vi "Init Aurora.vi"(8 "error in (no error)":errorcluster, 11 "Aurora COM Port":T1=enum."COM4") -> (0 "error out":errorcluster, 2 "Aurora Connected?":bool, 3 "Frame Grabber Data":T2)   [LabVIEW 2017]
uses:
  Controls/Tracking Data.ctl
  Controls/Packet Data.ctl
  Controls/Rigid Body Info.ctl
  Controls/Position.ctl
  Controls/Orientation.ctl
  Controls/Tracker Type.ctl
  Controls/COM Port.ctl
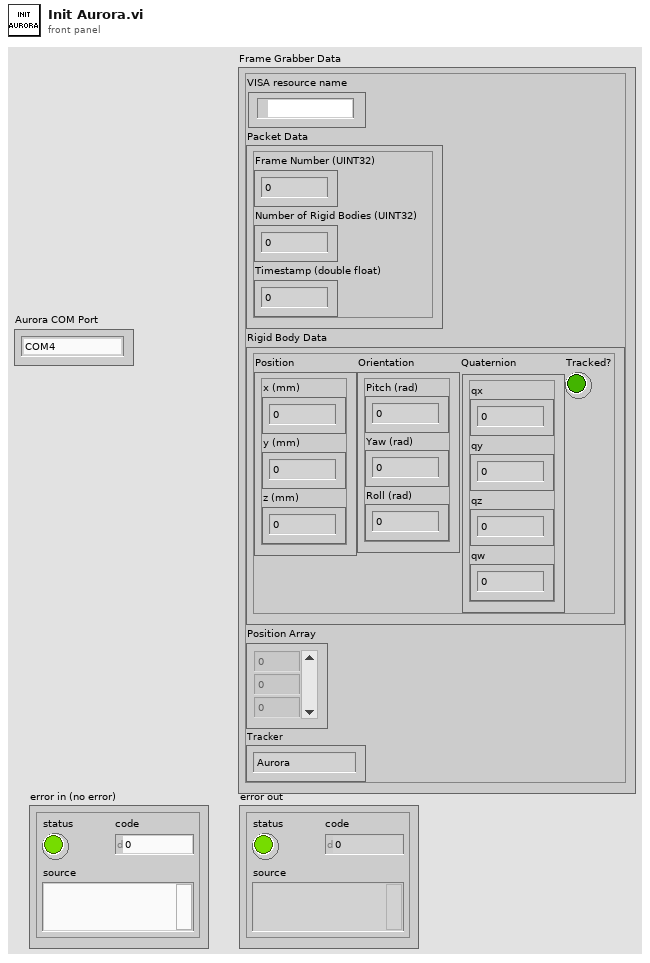
[diagram p1: front panel]
types:
  T1 = typedef "COM Port.ctl" = enum16{"COM1", "COM2", "COM3", "COM4", "COM5", "COM6", "COM7", "COM8", "COM9", "COM10", "COM11", "COM12", "COM13", "COM14", "COM15", "COM16", "COM17", "COM18", "COM19", "COM20"}
  T2 = typedef "Tracking Data.ctl" = cluster{"VISA resource name":refnum<visa-resource-name>, "Packet Data":T3, "Rigid Body Data":T4, "Position Array":dbl[][], "Tracker":T7}
  T3 = typedef "Packet Data.ctl" = cluster{"Frame Number (UINT32)":u32, "Number of Rigid Bodies (UINT32)":u32, "Timestamp (double float)":dbl}
  T4 = typedef "Rigid Body Info.ctl" = cluster{"Position":T5, "Orientation":T6, "Quaternion":cluster{"qx":sgl, "qy":sgl, "qz":sgl, "qw":sgl}, "Tracked?":bool}
  T5 = typedef "Position.ctl" = cluster{"x (mm)":sgl, "y (mm)":sgl, "z (mm)":sgl}
  T6 = typedef "Orientation.ctl" = cluster{"Pitch (rad)":sgl, "Yaw (rad)":sgl, "Roll (rad)":sgl}
  T7 = typedef "Tracker Type.ctl" = enum16{"Aurora", "OptiTrack"}
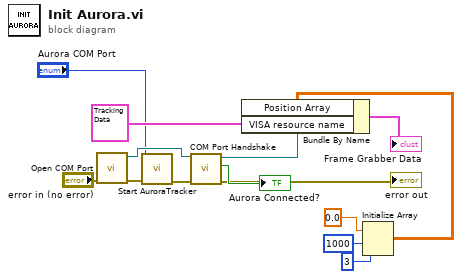
[diagram p0: block diagram]
diagram:
  n1 = call "Open COM Port.vi"("error in (no error)"="error in (no error)") -> ("error out"=w6:errorcluster, "VISA Refnum out"=w8:refnum<visa-resource-name>)  [unwired: 9 in]
  n2 = call "Start AuroraTracker.vi"("Error In"=w6, "Aurora COM Port"="Aurora COM Port") -> ("Error Out"=w7:errorcluster)  [unwired: 9 in]
  n3 = call "COM Port Handshake.vi"("error in (no error)"=w7, "VISA Refnum in"=w8) -> ("error out"=→"error out":errorcluster, "OptiTrack Connected?"=→"Aurora Connected?":bool, "VISA Refnum out"=w11:refnum<visa-resource-name>)  [unwired: 7 in]
  n4 = Initialize Array(0.0 ("element"), 1000 ("dimension size"), 3 ("dimension size")) -> (w2:dbl[][])
  n5 = Bundle By Name(cluster=T2 {"VISA resource name"="", "Packet Data"={"Frame Number (UINT32)"=0, "Number of Rigid Bodies (UINT32)"=0, "Timestamp (double float)"=0.0}, "Rigid Body Data"={"Position"={"x (mm)"=0.0, "y (mm)"=0.0, "z (mm)"=0.0}, "Orientation"={"Pitch (rad)"=0.0, "Yaw (rad)"=0.0, "Roll (rad)"=0.0}, "Quaternion"={"qx"=0.0, "qy"=0.0, "qz"=0.0, "qw"=0.0}, "Tracked?"=FALSE}, "Position Array"=[], "Tracker"=enum."Aurora"} ("Frame Grabber Data"), "Position Array"=w2, "VISA resource name"=w11) -> (→"Frame Grabber Data":T2)
